vi "Old Helium Fridge Cool-Down - With iTC and Fluke MM.vi"() -> ()   [LabVIEW 2014]
uses:
  <vilib>/Analysis/8numeric.llb/1D Numeric Integration.vi
  <instrlib>/Mercury iXX/Public/Libraries/System/Open/Open System.vi
  <vilib>/express/express shared/transition.llb/Dynamic To Waveform Array.vi
  <vilib>/express/express signal manip/GetorSetDDTAttributes/Set DDT Attributes/SetT0.vi
  <vilib>/express/express shared/transition.llb/Waveform Array To Dynamic.vi
  <vilib>/express/express signal manip/GetorSetDDTAttributes/Set DDT Attributes/Set DDT Properties.xnode
  <vilib>/Analysis/NI_AALPro.lvlib
  <instrlib>/Mercury iXX/Mercury iXX.lvlib
  <instrlib>/Mercury iXX/Public/Libraries/System.lvlib
panel:
  out "Centroid:":dbl
  out "Tri":bool
  out "NMR":bool
  out "NMR":cluster{"Y":dbl[], "Y":dbl[]}[](graph)
  out "AB4.R":dynamicdata(graph)
  out "AB4.T":dynamicdata(graph)
  out "AB3.R":dynamicdata(graph)
  out "AB3.T":dynamicdata(graph)
  out "Fluke Err":bool
  out "Mag. Field (T)":dbl
  in  "Peak Location (MHz)":dbl
  in  "Baseline Subtract":bool
  out "AB2.R":dynamicdata(graph)
  out "AB2.T":dynamicdata(graph)
  out "Peak Location (MHz)":dbl
  in  "Mag. Field (T)":dbl
  out "i":dbl
  in  "VISA resource name":refnum<visa-resource-name>="MERCURYITC"
  in  "Time b/t iTC Resets\n(min)":dbl=45.0
  out "Time Since iTC Reset\n(min)":dbl
  out "iTC Last Reset":timestamp
  out "Reset iTC":bool
  in  "Wing Fit Poly":i32=3 min=0 max=4 step=1
  out "Just Started":bool
  out "Up/Down Ave Y Final":dbl[](array[numeric])
  in  "Use Wing Fit":bool=TRUE
  out "Triangle Wave\nRate (Hz)":dbl
  in  "NMR Temp Points/Measurement":dbl=20.0
  in  "Peak Size":dbl=15.0 min=0.0 max=100.0
  out "Wing Fit":dbl[](array[numeric])
  out "Fit Y":dbl[](array[numeric])
  out "Fit X":dbl[](array[numeric])
  in  "Wing Size (%)":dbl=20.0 min=0.0 max=100.0
  out "Normalized\nAdditive NMR Y":dbl[](array[numeric])
  out "Up/Down Ave Y":dbl[](array[numeric])
  out "Up/Down Ave X":dbl[](array[numeric])
  out "Baseline\nSubtract":bool
  out "Depth/Div Submit":bool
  out "Cent. Frq. Submit":bool
  out "Insta Mod One":dbl[](array[numeric])
  out "Insta Tri":dbl[](array[numeric])
  out "Insta Mod Sweeps":dbl[](array[numeric])
  in  "Triangle Wave Rate\nSubmit":bool
  in  "Session In 3":refnum<visa-resource-name>="HPSIGGEN"
  in  "error in 3":errorcluster {"code" format="%.0x"}
  out "Central Frequency 2":dbl
  out "error out 3":errorcluster {"code" format="%.0x"}
  out "Session Out 3":refnum<visa-resource-name>
  out "Reset Sweep":bool
  out "Add Mod Sweep":dbl[](array[numeric])
  out "Sweep Iter":i32
  out "Array Size":i32
  out "Modulator":dbl[](array[numeric])
  out "Reference Triangle Wave":dbl[](array[numeric])
  out "Input Triangle Wave":dbl[](array[numeric])
  out "Triangle Check":dbl
  out "NMR X Check":dbl[](array[numeric])
  out "NMR":cluster{"Y":dbl[], "Y":dbl[]}[](graph)
  in  "Reset Total\nSweeps":bool
  out "Number of Total\nSweeps Added":i32
  out "Additive NMR Y":dbl[](array[numeric])
  out "Good NMR X":dbl[](array[numeric])
  in  "Record All\nSweep Sets":bool
  out "Flow (SLM)":dbl
  out "NMR":bool
  out "AB   .T":i32
  out "AB":i32
  out "Roots Flow (SLM)":dynamicdata(graph)
  in  "DV4/DV6":bool
  out "Temp":bool
  out "AB5.R":dynamicdata(graph)
  out "CCS.R":dynamicdata(graph)
  out "AB2/3/4.R":dynamicdata(graph)
  out "AB1.R":dynamicdata(graph)
  out "AB5.T":dynamicdata(graph)
  out "CCS.T":dynamicdata(graph)
  out "AB2/3/4.T":dynamicdata(graph)
  out "AB1.T":dynamicdata(graph)
  out "Vapor Pressure\n(mTorr)":dbl
  out "V.P. Voltage\n(V)":dbl
  in  "LN2/LHe":bool=TRUE
  out "V.P. Temp\n(K)":dbl
  out "Vapor Pressure":dynamicdata(graph)
  out "Vapor Pressure\n(mbar)":dbl format="%#_3e"
  out "Vapor Pressure\n(mTorr)":dbl
  in  "Time Between\nTemp Ponts (s)":dbl=5.0
  out "?":dbl
  out "?":dbl
  out "?":dbl
  out "?":dbl
  out "Baseline X":dbl[](array[numeric])
  out "Session Out 2":refnum<visa-resource-name>
  out "error out 2":errorcluster {"code" format="%.0x"}
  out "token":dbl
  in  "error in 2":errorcluster {"code" format="%.0x"}
  in  "Session In 2":refnum<visa-resource-name>="HPSIGGEN"
  in  "Depth/Div Submit":bool
  out "Depth/Div (kHz)":dbl
  in  "Cent. Frq. Submit":bool
  out "Session Out":refnum<visa-resource-name>
  out "error out":errorcluster {"code" format="%.0x"}
  out "Central Frequency":dbl
  in  "error in":errorcluster {"code" format="%.0x"}
  in  "Session In":refnum<visa-resource-name>="HPSIGGEN"
  out "Cent. Freq. (MHz)":dbl
  out "Temp":bool
  out "Temperature Strip Chart":dynamicdata(graph)
  out "Q Meter Temp":dynamicdata(graph)
  out "Zeroed Array":dbl[](array[numeric])
  in  "Submit":bool
  out "Is Flashing":bool
  in  "Error Beat":bool
  in  "Clear":bool
  in  "Comment":string
  out "Heartbeat":bool
  out "Most Recent Error":string
  out "Baseline Subtracted Integral vs. Time":dbl(graph)
  out "Time of Last Baseline":string
  out "Baseline Y":dbl[](array[numeric])
  in  "Get Baseline":bool
  out "Recording":bool
  out "Time of Last Recording":string
  in  "Record Next \nSweep Set":bool
  in  "Depth/Div\n(MHz)":dbl=0.5
  in  "Central Freq. \n(MHz)":dbl=12.996
  in  "Triangle Wave\nRate (Hz)":dbl=15.862
  out "Time Elapsed \nDuring Sweeps (s)":dbl
  out "Lab Time":string
  out "Most Recent Error (NMR)":string
  out "Last Sweep Start Time":string
  out "Most Recent Error (Temp)":string
  out "Last Measurement Taken":string
  out "VI Start Time":string
  out "Temp":bool
  out "NMR":bool
  in  "stop":bool
  out "Input Triangle Wave":dynamicdata(graph)
  out "Modulator":dynamicdata(graph)
  in  "# of Sweeps":i32=1
  out "Resistance Strip Chart":dynamicdata(graph)
  in  "Heartbeat":bool
  in  "Temp Strip Chart":bool
  out "Errors":bool
  in  "Silence Flashing":bool
  in  "Ignore \nErrors":bool
  out "NMR":cluster{"Y":dbl[], "Y":dbl[]}[](graph)
  in  "AB2/3/4 Switch":T1(radio)=enum."Radio Selection 3"
  # "Initialization and Logic Controls -- DO NOT TOUCH!!"
  # "Signal Generator Logic -- DO NOT TOUCH!!"
  # "To Clean and Get Rid Of"
  # "Baseline = 3000 Sweeps"
  # "TE > 2000 Sweeps"
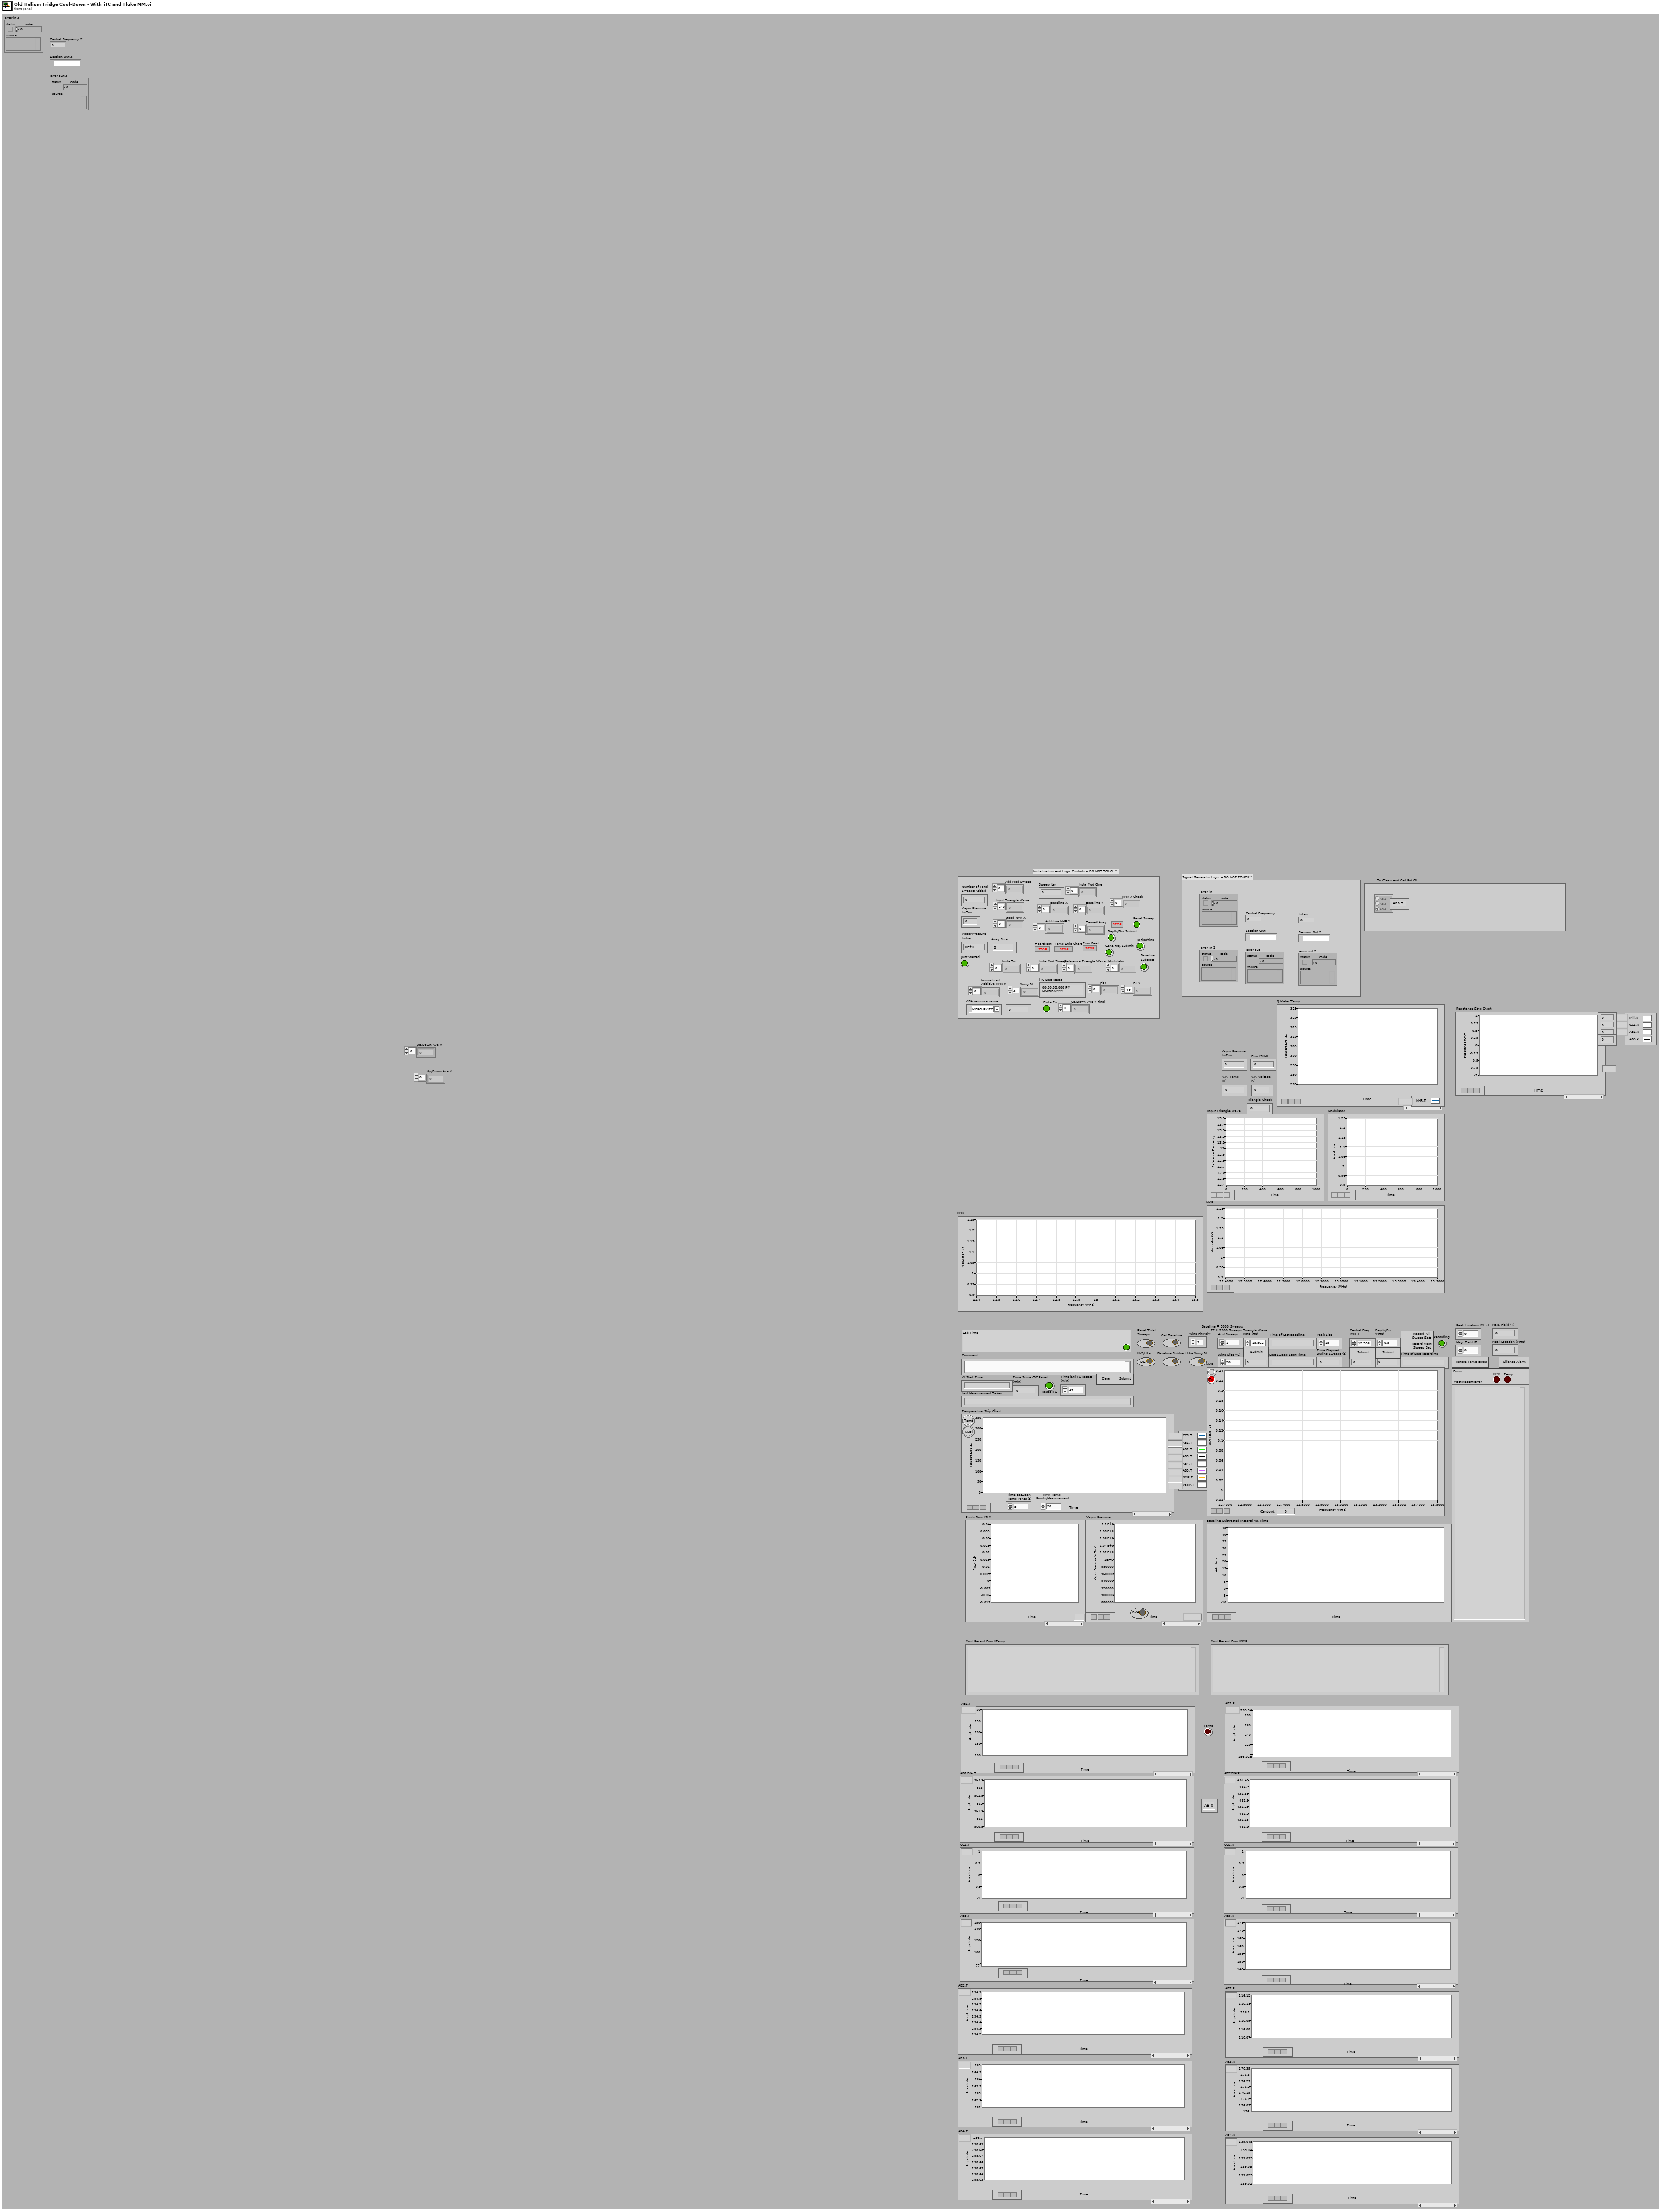
[diagram p1: front panel]
types:
  T1 = enum32{"Radio Selection 1", "Radio Selection 2", "Radio Selection 3"}
  T2 = typedef "Mercury iXX.lvlib/Mercury Reference.ctl" = cluster{"Comms":refnum<visa-resource-name>, "Device ID":string[], "Comms Layer":T3, "Command":string, "Query reference":T4}
  T3 = typedef "Mercury iXX.lvlib/Comms Transport Layer.ctl" = enum16{"Ethernet TCP/IP", "USB", "ISOBus - RS-232", "GPIB"}
  T4 = typedef "Mercury iXX.lvlib/Query Dynamic Reference.ctl" = refnum<vi>
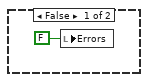
[diagram p2: hidden frame]
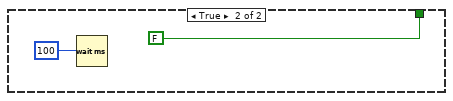
[diagram p4: hidden frame]
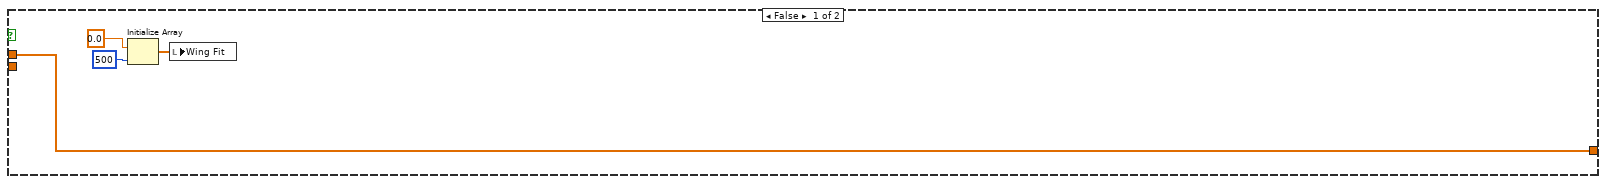
[diagram p6: hidden frame]
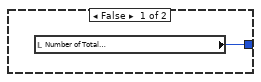
[diagram p8: hidden frame]
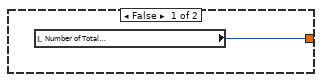
[diagram p10: hidden frame]
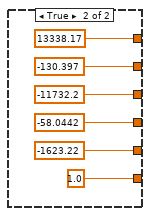
[diagram p11: hidden frame]
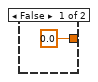
[diagram p12: hidden frame]
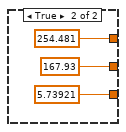
[diagram p13: hidden frame]
diagram:
  # "Initialize Baseline to All Zeros"
  n1 = while "NMR System" {
    stop <- "stop" stop-if-true
    w78 = 490
    w86 = 0
    w74 = 2.0
    w77 = 500
    n2 = local read "Just Started"() -> (w33:bool)
    n3 = local read "Just Started"() -> (w36:bool)
    n4 = local read "Just Started"() -> (w28:bool)
    n5 = local read "Central Frequency"() -> (w155:dbl)
    n6 = Get Date/Time In Seconds() -> (seconds since 1Jan1904=w171:timestamp)
    n7 = Or(x="Cent. Frq. Submit", y=w36) -> (x .or. y?=w34:bool)
    "Cent. Frq. Submit" <- w34
    n8 = Or(x="Triangle Wave Rate\nSubmit", y=w33) -> (x .or. y?=w31:bool)
    n9 = Or(x="Depth/Div Submit", y=w28) -> (x .or. y?=w29:bool)
    "Depth/Div Submit" <- w29
    n10 = Get Date/Time String(seconds (now)=w171, want seconds? (F)=TRUE) -> (date string=w174:string, time string=w176:string)  [unwired: 1 in]
    n11 = case "Set Central Frequency" shown="True" w34 {
      tunnel: "Central Freq. \n(MHz)" -> [_ w353]
      frame False {
      }
      frame True {
        w351 = " MHz; FREQuency:CW?"  # Command
        w354 = "FREQuency "  # Command
        w372 = "[,;\r\n\t]+"  # Delimiters
        w369 = "%.;%f"  # Format String
        (unwired) "FREQuency 12.996 MHz; FREQuency:CW?"  # Command
        w360 = u8 0  # Termination Char
        w355 = u32 3000  # Timeout
        # "Parse the output text based on the Format String"
        # "Perform a VISA Write and Read (Query)"
        # "Keep reading 4096 bytes while the error returned from the\nVISA read 0x3FFF0006 (there's more data in the buffer to read)."
        # "Set the termination character"
        n12 = property class="Instr"(reference="Session In", error in="error in", "General Settings:Timeout Value"=w355) -> (reference out=w361:refnum<visa-resource-name>, error out=w358:errorcluster)
        n13 = property class="Instr"(reference=w361, error in=w358, "Message Based Settings:Termination Character"=w360, "Message Based Settings:Termination Character Enable"=FALSE ("enable")) -> (reference out=w373:refnum<visa-resource-name>, error out=w359:errorcluster)
        "Session Out" <- w373
        n14 = Number To Fractional String(number=w353) -> (F-format string=w352:string)  [unwired: 3 in]
        n15 = Concatenate Strings(w354, w352, w351) -> (w350:string)
        n16 = VISA Write(VISA resource name=w373, write buffer=w350, error in (no error)=w359) -> (VISA resource name out=w363:refnum<visa-resource-name>, error out=w364:errorcluster)  [unwired: 1 out]
        n17 = while {
          tunnel: w363 -> [w380]
          shift-right: [w374] -> w367
          shift-left: "" -> [w379]
          tunnel: w364 -> [w377]
          tunnel: [w376] -> w365
          stop <- w375 continue-if-true
          n18 = VISA Read(VISA resource name=w380, byte count=u32 4096 ("byte count (0)"), error in (no error)=w377) -> (read buffer=w378:string, error out=w376:errorcluster)  [unwired: 2 out]
          n19 = Unbundle By Name(w376) -> ("code"=w382:i32)
          n20 = Concatenate Strings(w379, w378) -> (w374:string)
          n21 = Equal?(x=1073676294, y=w382) -> (x = y?=w375:bool)
        }
        n22 = Match Pattern(string=w367, regular expression=w372) -> (before substring=w368:string)  [unwired: 1 in, 3 out]
        n23 = Scan From String(format string=w369, input string=w368, error in=w365) -> (error out=→"error out":errorcluster, output 1=→"Central Frequency":dbl)  [unwired: 2 in, 2 out]
      }
    }
    n24 = case "Set Triangle Wave Frequency" shown="True" w31 {
      tunnel: "Triangle Wave\nRate (Hz)" -> [_ w235]
      frame False {
      }
      frame True {
        w237 = " Hz; FM1:INTernal:FREQuency?"  # Command
        w239 = "FM1:INTernal1:FREQuency "  # Command
        w256 = "[,;\r\n\t]+"  # Delimiters
        w254 = "%.;%f"  # Format String
        (unwired) "FM1:INTernal1:FREQuency 15 Hz; FM1:INTernal:FREQuency?"  # Command
        w245 = u8 0  # Termination Char
        w240 = u32 3000  # Timeout
        # "Parse the output text based on the Format String"
        # "Perform a VISA Write and Read (Query)"
        # "Keep reading 4096 bytes while the error returned from the\nVISA read 0x3FFF0006 (there's more data in the buffer to read)."
        # "Set the termination character"
        n25 = property class="Instr"(reference="Session In 3", error in="error in 3", "General Settings:Timeout Value"=w240) -> (reference out=w246:refnum<visa-resource-name>, error out=w243:errorcluster)
        n26 = property class="Instr"(reference=w246, error in=w243, "Message Based Settings:Termination Character"=w245, "Message Based Settings:Termination Character Enable"=FALSE ("enable")) -> (reference out=w257:refnum<visa-resource-name>, error out=w244:errorcluster)
        "Session Out 3" <- w257
        n27 = Number To Fractional String(number=w235) -> (F-format string=w238:string)  [unwired: 3 in]
        n28 = Concatenate Strings(w239, w238, w237) -> (w236:string)
        n29 = VISA Write(VISA resource name=w257, write buffer=w236, error in (no error)=w244) -> (VISA resource name out=w248:refnum<visa-resource-name>, error out=w249:errorcluster)  [unwired: 1 out]
        n30 = while {
          tunnel: w248 -> [w264]
          shift-right: [w258] -> w252
          shift-left: "" -> [w263]
          tunnel: w249 -> [w261]
          tunnel: [w260] -> w250
          stop <- w259 continue-if-true
          n31 = VISA Read(VISA resource name=w264, byte count=u32 4096 ("byte count (0)"), error in (no error)=w261) -> (read buffer=w262:string, error out=w260:errorcluster)  [unwired: 2 out]
          n32 = Unbundle By Name(w260) -> ("code"=w266:i32)
          n33 = Concatenate Strings(w263, w262) -> (w258:string)
          n34 = Equal?(x=1073676294, y=w266) -> (x = y?=w259:bool)
        }
        n35 = Match Pattern(string=w252, regular expression=w256) -> (before substring=w253:string)  [unwired: 1 in, 3 out]
        n36 = Scan From String(format string=w254, input string=w253, error in=w250) -> (error out=→"error out 3":errorcluster, output 1=→"Central Frequency 2":dbl)  [unwired: 2 in, 2 out]
        "Triangle Wave\nRate (Hz)" <- w235
      }
    }
    n37 = local read "token"() -> (w152:dbl)
    n38 = case "Set Depth/Div" shown="True" w29 {
      tunnel: "Depth/Div\n(MHz)" -> [_ w315]
      frame False {
      }
      frame True {
        w317 = " Hz; :FM1:DEViation?"  # Command
        w322 = "[,;\r\n\t]+"  # Delimiters
        w325 = "%.;%f"  # Format String
        w319 = ":FM1:DEViation "  # Command
        w334 = u8 0  # Termination Char
        w339 = u32 3000  # Timeout
        # "Parse the output text based on the Format String"
        # "Perform a VISA Write and Read (Query)"
        # "Keep reading 4096 bytes while the error returned from the\nVISA read 0x3FFF0006 (there's more data in the buffer to read)."
        # "Set the termination character"
        n39 = property class="Instr"(reference="Session In 2", error in="error in 2", "General Settings:Timeout Value"=w339) -> (reference out=w333:refnum<visa-resource-name>, error out=w336:errorcluster)
        n40 = Multiply(x=w315, y=1000000.0) -> (x*y=w314:dbl)
        n41 = property class="Instr"(reference=w333, error in=w336, "Message Based Settings:Termination Character"=w334, "Message Based Settings:Termination Character Enable"=FALSE ("enable")) -> (reference out=w321:refnum<visa-resource-name>, error out=w335:errorcluster)
        "Session Out 2" <- w321
        n42 = Number To Fractional String(number=w314) -> (F-format string=w318:string)  [unwired: 3 in]
        n43 = Concatenate Strings(w319, w318, w317) -> (w320:string)
        n44 = VISA Write(VISA resource name=w321, write buffer=w320, error in (no error)=w335) -> (VISA resource name out=w331:refnum<visa-resource-name>, error out=w330:errorcluster)  [unwired: 1 out]
        n45 = while {
          tunnel: w331 -> [w346]
          shift-right: [w340] -> w327
          shift-left: "" -> [w345]
          tunnel: w330 -> [w343]
          tunnel: [w342] -> w329
          stop <- w341 continue-if-true
          n46 = VISA Read(VISA resource name=w346, byte count=u32 4096 ("byte count (0)"), error in (no error)=w343) -> (read buffer=w344:string, error out=w342:errorcluster)  [unwired: 2 out]
          n47 = Unbundle By Name(w342) -> ("code"=w348:i32)
          n48 = Concatenate Strings(w345, w344) -> (w340:string)
          n49 = Equal?(x=1073676294, y=w348) -> (x = y?=w341:bool)
        }
        n50 = Match Pattern(string=w327, regular expression=w322) -> (before substring=w326:string)  [unwired: 1 in, 3 out]
        n51 = Scan From String(format string=w325, input string=w326, error in=w329) -> (error out=→"error out 2":errorcluster, output 1=→"token":dbl)  [unwired: 2 in, 2 out]
      }
    }
    n52 = Concatenate Strings(w174, " ", w176) -> (w166:string)
    n53 = Divide(x=w155, y=1000000.0) -> (x/y=w154:dbl)
    "Cent. Freq. (MHz)" <- w154
    n54 = Divide(x=w152, y=1000000.0) -> (x/y=w151:dbl)
    "Depth/Div (kHz)" <- w151
    n55 = while "Sweep-Averaged Modulator and Triangle Input" {
      tunnel: "# of Sweeps" -> [w585]
      tunnel: 1000 -> [w555]
      tunnel: [w568] -> w93
      tunnel: w166 -> [w595]
      tunnel: [w594] -> w172
      tunnel: [w593] -> w169
      tunnel: w151 -> [w589]
      tunnel: w154 -> [w587]
      tunnel: [w586] -> w94
      tunnel: [w580] -> w158
      tunnel: [w575] -> w140
      tunnel: [w569] -> w103
      i -> [w570]
      stop <- w556 stop-if-true
      w550 = 42.57
      w583 = 0.0
      n56 = local read "Reset Sweep"() -> (w557:bool)
      n57 = local read "Sweep Iter"() -> (w560:i32)
      n58 = Greater Or Equal?(x=w570, y=w585) -> (x >= y?=w558:bool)
      n59 = Equal To 0?(x=w570) -> (x = 0?=w564:bool)
      n60 = local read "Triangle Wave\nRate (Hz)"() -> (w554:dbl)
      n61 = Multiply(x="Mag. Field (T)", y=w550) -> (x*y=→"Peak Location (MHz)":dbl)
      n62 = Not Equal To 0?(x=w560) -> (x != 0?=w561:bool)
      n63 = case shown="True" w564 {
        frame False {
        }
        frame True {
          "Sweep Iter" <- 0
        }
      }
      n64 = Compound Arithmetic op=OR(w558, w557) -> (w556:bool)
      n65 = Divide(x="Peak Location (MHz)", y=w550) -> (x/y=→"Mag. Field (T)":dbl)
      n66 = case shown="True" w561 {
        frame False {
        }
        frame True {
          n67 = control-ref of="Reference Triangle Wave"() -> (w613:refnum<vi>)
          n68 = local read "Baseline\nSubtract"() -> (w608:bool)
          n69 = control-ref of="Insta Mod Sweeps"() -> (w615:refnum<vi>)
          n70 = control-ref of="Number of Total\nSweeps Added"() -> (w606:refnum<vi>)
          n71 = control-ref of="Up/Down Ave X"() -> (w602:refnum<vi>)
          n72 = control-ref of="Normalized\nAdditive NMR Y"() -> (w607:refnum<vi>)
          n73 = control-ref of="Insta Mod One"() -> (w609:refnum<vi>)
          n74 = control-ref of="Baseline X"() -> (w610:refnum<vi>)
          n75 = control-ref of="Baseline Y"() -> (w611:refnum<vi>)
          n76 = control-ref of="Sweep Iter"() -> (w612:refnum<vi>)
          n77 = control-ref of="Insta Tri"() -> (w614:refnum<vi>)
          n78 = control-ref of="Fit X"() -> (w605:refnum<vi>)
          n79 = control-ref of="Fit Y"() -> (w604:refnum<vi>)
          n80 = control-ref of="Wing Fit"() -> (w603:refnum<vi>)
          n81 = control-ref of="Up/Down Ave Y"() -> (w601:refnum<vi>)
          n82 = call "Baseline Monitor.vi"("Baseline X"=w610, "Baseline Y"=w611, "Sweep Iter"=w612, "Reference Triangle Wave"=w613, "Input Triangle Wave"=w614, "Modulator"=w615, "Insta Mod"=w609, "Normalized\nAdditive NMR\nY"=w607, "Baseline\nSubtract"=w608, "Wings X"=w605, "# of Sweeps"=w606, "Wings Y"=w604, "Wing Fit"=w603, "Up/Down Ave X"=w602, "Up/Down Ave Y"=w601) -> ()  [unwired: 5 in]
        }
      }
      n83 = To Double Precision Float(number=w555) -> (double precision float=w592:dbl)
      n84 = Multiply(x=w554, y=w592) -> (x*y=w553:dbl)
      n85 = call "Get NMR Data"("rate"=w553, "number of samples"=w555) -> ("data"=w600:dynamicdata, "error out"=w575:errorcluster)  [unwired: 15 in, 1 out]
      n86 = while {
        tunnel: ["NMR Temp Points/Measurement"] -> w578
        tunnel: [w646] -> w577
        tunnel: w575 -> [w642]
        i -> [w645]
        stop <- w644 stop-if-true
        n87 = call "Get NMR Temp"("error in"=w642) -> ("data"=w648:dynamicdata)  [unwired: 16 in, 2 out]
        n88 = Add(x=w648, y=273.15) -> (x+y=w647:dynamicdata)
        n89 = call "Convert from Dynamic Data7"("Dynamic Data Type"=w647) -> ("Scalar"=w650:dbl)  [unwired: 3 in]
        n90 = Equal To 0?(x=w645) -> (x = 0?=w651:bool)
        n91 = Greater Or Equal?(x=w645, y="NMR Temp Points/Measurement") -> (x >= y?=w644:bool)
        n92 = feedback #1() -> (w653:dbl)  [unwired: 1 in]
        n93 = Add(x=w650, y=w653) -> (x+y=w646:dbl)
        n94 = Select(t=0.0, s=w651, f=w646) -> (s? t:f=w652:dbl)
        n95 = feedback-in #1(w652) -> ()
      }
      n96 = Split Signals(w600) -> (w591:dynamicdata, w599:dynamicdata)  [unwired: 2 in]
      n97 = call <vilib>:"General Error Handler.vi"("type of dialog (OK msg:1)"=0, "error in (no error)"=w575) -> ("error?"=w579:bool, "message"=w597:string, "error out"=w593:errorcluster)  [unwired: 9 in, 2 out]
      "NMR" <- w579
      "NMR" <- w579
      n98 = call "Convert from Dynamic Data2"("Dynamic Data Type"=w591) -> ("Array"=w590:dbl[])  [unwired: 3 in]
      n99 = call "Convert from Dynamic Data"("Dynamic Data Type"=w599) -> ("Array"=w559:dbl[])  [unwired: 3 in]
      "Insta Mod One" <- w559
      n100 = case shown="False" w579 {
        tunnel: w597 -> [_ w657]
        tunnel: w595 -> [w655 _]
        frame False {
          "Last Sweep Start Time" <- w655
        }
        frame True {
          n101 = local read "Lab Time"() -> (w659:string)
          n102 = Concatenate Strings(w659, "; ", w657) -> (→"Most Recent Error (NMR)":string)
        }
      }
      n103 = Multiply(x=w590, y=w589) -> (x*y=w588:dbl[])
      n104 = Add(x=w588, y=w587) -> (x+y=w562:dbl[])
      "Insta Tri" <- w562
      n105 = local read "Good NMR X"() -> (w574:dbl[])
      n106 = while {
        tunnel: w562 -> [w627]
        tunnel: w574 -> [w626]
        tunnel: [w624] -> w572
        i -> [w623]
        stop <- w637 stop-if-true
        n107 = Array Size(array=w627) -> (size(s)=w624:i32)
        n108 = Greater Or Equal?(x=w623, y=w624) -> (x >= y?=w637:bool)
        n109 = Equal To 0?(x=w623) -> (x = 0?=w630:bool)
        n110 = Index Array(array=w626, index=w623) -> (element=w625:dbl)
        n111 = case shown="True" w630 {
          frame False {
          }
          frame True {
            "Triangle Check" <- 0.0
          }
        }
        n112 = Multiply(x=0.01, y=w625) -> (x*y=w634:dbl)
        n113 = Add(x=w634, y=w625) -> (x+y=w635:dbl)
        n114 = Subtract(x=w625, y=w634) -> (x-y=w633:dbl)
        n115 = Index Array(array=w627, index=w623) -> (element=w628:dbl)
        n116 = Less?(x=w628, y=w635) -> (x < y?=w632:bool)
        n117 = Greater?(x=w628, y=w633) -> (0:w631:bool)
        n118 = And(x=w632, y=w631) -> (x .and. y?=w629:bool)
        n119 = case shown="True" w629 {
          frame False {
          }
          frame True {
            n120 = local read "Triangle Check"() -> (w639:dbl)
            n121 = Add(x=1.0, y=w639) -> (x+y=w640:dbl)
            n122 = local write "Triangle Check"(w640) -> ()
          }
        }
      }
      "Array Size" <- w572
      n123 = call "Convert to Dynamic Data10"("Array"=w562) -> ("Dynamic Data Type"=w586:dynamicdata)  [unwired: 3 in]
      n124 = local read "Sweep Iter"() -> (w569:i32)
      n125 = Divide(x=w577, y=w578) -> (x/y=w576:dbl)
      n126 = local read "Add Mod Sweep"() -> (w565:dbl[])
      n127 = Initialize Array(w583, w555) -> (w598:dbl[])
      n128 = Equal To 0?(x=w569) -> (x = 0?=w584:bool)
      n129 = local read "Sweep Iter"() -> (w566:i32)
      n130 = Select(t=w598, s=w584, f=w565) -> (s? t:f=w567:dbl[])
      "Add Mod Sweep" <- w567
      n131 = feedback #2() -> (w581:dbl)  [unwired: 1 in]
      n132 = Add(x=w576, y=w581) -> (x+y=w580:dbl)
      n133 = Select(t=w583, s=w584, f=w580) -> (s? t:f=w582:dbl)
      n134 = feedback-in #2(w582) -> ()
      n135 = Divide(x=w567, y=w566) -> (x/y=→"Insta Mod Sweeps":dbl[])
      n136 = local read "Triangle Check"() -> (w573:dbl)
      n137 = Equal?(x=w573, y=w572) -> (x = y?=w571:bool)
      "Tri" <- w571
      n138 = case shown="True" w571 {
        tunnel: w559 -> [_ w620]
        frame False {
        }
        frame True {
          n139 = local read "Sweep Iter"() -> (w618:i32)
          n140 = local read "Add Mod Sweep"() -> (w621:dbl[])
          n141 = Add(x=w618, y=1) -> (x+y=w616:i32)
          n142 = Add(x=w621, y=w620) -> (x+y=w619:dbl[])
          n143 = local write "Sweep Iter"(w616) -> ()
          n144 = local write "Add Mod Sweep"(w619) -> ()
        }
      }
      n145 = local read "Add Mod Sweep"() -> (w568:dbl[])
      n146 = Get Date/Time In Seconds() -> (seconds since 1Jan1904=w594:timestamp)
    }
    n147 = local read "Good NMR X"() -> (w110:dbl[])
    n148 = local read "Depth/Div Submit"() -> (w98:bool)
    n149 = local read "Cent. Frq. Submit"() -> (w99:bool)
    n150 = local read "Just Started"() -> (w37:bool)
    n151 = call "Convert to Dynamic Data33"("Array"=w110) -> ("Dynamic Data Type"=w105:dynamicdata)  [unwired: 3 in]
    n152 = call "DAQ Assistant"("error in"=w140) -> ("data"=w146:dynamicdata, "error out"=w130:errorcluster)  [unwired: 16 in, 1 out]
    n153 = case shown="False" "DV4/DV6" {
      tunnel: [9.563177 13338.17] -> w139
      tunnel: [-6.30995 -130.397] -> w138
      tunnel: [-4.4943 -11732.2] -> w137
      tunnel: [-6.91233 -58.0442] -> w136
      tunnel: [-5.10184 -1623.22] -> w135
      tunnel: [1000.0 1.0] -> w133
      frame False {
      }
      frame True {
      }
    }
    n154 = case shown="False" w37 {
      selector: w37 -> [w179 _]
      tunnel: [w179 FALSE] -> w27
      frame False {
      }
      frame True {
        n155 = Wait (ms)(milliseconds to wait=100) -> ()  [unwired: 1 out]
      }
    }
    n156 = Subtract(x=w172, y=w171) -> (x-y=→"Time Elapsed \nDuring Sweeps (s)":dbl)
    n157 = Merge Signals(w94, w105) -> (→"Input Triangle Wave":dynamicdata)
    n158 = call "Convert from Dynamic Data9"("Dynamic Data Type"=w105) -> ("Array"=→"Reference Triangle Wave":dbl[])  [unwired: 3 in]
    n159 = Compound Arithmetic op=OR(w37, "Reset Total\nSweeps", w99, w98) -> (w100:bool)
    "Reset Sweep" <- w100
    n160 = call "Convert from Dynamic Data8"("Dynamic Data Type"=w94) -> ("Array"=w107:dbl[])  [unwired: 3 in]
    "Input Triangle Wave" <- w107
    n161 = Divide(x=w93, y=w103) -> (x/y=w68:dbl[])
    "Modulator" <- w68
    n162 = Divide(x=w158, y=w103) -> (x/y=w159:dbl)
    n163 = local read "Tri"() -> (w104:bool)
    n164 = case shown="True" w104 {
      tunnel: w93 -> [_ w272]
      tunnel: [w268 w270] -> w109
      tunnel: w103 -> [_ w269]
      frame False {
        n165 = local read "Number of Total\nSweeps Added"() -> (w268:i32)
      }
      frame True {
        n166 = local read "Additive NMR Y"() -> (w274:dbl[])
        n167 = local read "Number of Total\nSweeps Added"() -> (w271:i32)
        n168 = Add(x=w272, y=w274) -> (x+y=w273:dbl[])
        n169 = local write "Additive NMR Y"(w273) -> ()
        n170 = Add(x=w271, y=w269) -> (x+y=w270:i32)
      }
    }
    "Number of Total\nSweeps Added" <- w109
    n171 = case shown="True" w100 {
      tunnel: w107 -> [_ w275]
      frame False {
      }
      frame True {
        n172 = local write "Good NMR X"(w275) -> ()
      }
    }
    n173 = case shown="True" w100 {
      tunnel: [w276 0.0] -> w64
      frame False {
        n174 = local read "Number of Total\nSweeps Added"() -> (w276:i32)
      }
      frame True {
        n175 = Initialize Array(0.0, 1000) -> (w277:dbl[])
        n176 = local write "Good NMR X"(w277) -> ()
        n177 = local write "Additive NMR Y"(w277) -> ()
      }
    }
    n178 = call "DAQ Assistant2"("error in"=w130) -> ("data"=w129:dynamicdata)  [unwired: 16 in, 2 out]
    n179 = local read "Baseline Y"() -> (w79:dbl[])
    n180 = Add(x=w78, y=w77) -> (x+y=w85:i32)
    n181 = Greater Than 0?(x=w159) -> (x > 0?=w165:bool)
    n182 = To Double Precision Float(number=w146) -> (double precision float=w141:dbl)
    "V.P. Voltage\n(V)" <- w141
    n183 = Less?(x=w159, y=500.0) -> (x < y?=w162:bool)
    n184 = To Double Precision Float(number=w129) -> (double precision float=w128:dbl)
    n185 = Array Subset(array=w68, index=w78, length=w77) -> (w97:dbl[])
    n186 = Array Subset(array=w68, index=w85, length=w77) -> (w90:dbl[])
    n187 = call "Convert to Dynamic Data9"("Array"=w68) -> ("Dynamic Data Type"=w112:dynamicdata)  [unwired: 3 in]
    n188 = Array Subset(array=w79, index=w85, length=w77) -> (w84:dbl[])
    n189 = And(x=w162, y=w165) -> (x .and. y?=w164:bool)
    n190 = call "Convert to Dynamic Data15"("Double"=w159) -> ("Dynamic Data Type"=w160:dynamicdata)  [unwired: 3 in]
    n191 = Greater?(x=w141, y=0.049) -> (0:w145:bool)
    n192 = case "Take Baseline Structure" shown="True" "Get Baseline" {
      tunnel: w112 -> [_ w393]
      tunnel: w166 -> [_ w394]
      tunnel: w94 -> [_ w391]
      frame False {
      }
      frame True {
        n193 = call "Convert from Dynamic Data4"("Dynamic Data Type"=w393) -> ("Array"=w395:dbl[])  [unwired: 3 in]
        n194 = call "Convert from Dynamic Data6"("Dynamic Data Type"=w391) -> ("Array"=w392:dbl[])  [unwired: 3 in]
        n195 = local write "Baseline Y"(w395) -> ()
        n196 = local write "Baseline X"(w392) -> ()
        "Time of Last Baseline" <- w394
      }
    }
    n197 = case shown="True" w164 {
      tunnel: w160 -> [_ w384]
      frame False {
      }
      frame True {
        "Q Meter Temp" <- w384
      }
    }
    n198 = formula code="P=(a+c*V+e*V*V)/(1+b*V+d*V*V);"("V"=w141, "a"=w135, "b"=w136, "c"=w137, "d"=w138, "e"=w139) -> ("P"=w143:dbl)
    n199 = local write "Just Started"(w27) -> ()
    n200 = Array Size(array=w90) -> (size(s)=w89:i32)
    n201 = Array Subset(array=w68, index=w86, length=w78) -> (w92:dbl[])
    n202 = Array Size(array=w84) -> (size(s)=w83:i32)
    n203 = Array Subset(array=w79, index=w86, length=w78) -> (w82:dbl[])
    n204 = Not(x=w164) -> (.not. x?=→"NMR":bool)
    n205 = Multiply(x=w128, y=10.0) -> (x*y=w126:dbl)
    "Flow (SLM)" <- w126
    n206 = Insert Into Array(array=w90, index=w89, new element=w92) -> (w91:dbl[])
    n207 = Insert Into Array(array=w84, index=w83, new element=w82) -> (w81:dbl[])
    n208 = call "Convert to Dynamic Data20"("Double"=w126) -> ("Dynamic Data Type"=→"Roots Flow (SLM)":dynamicdata)  [unwired: 3 in]
    n209 = Select(t=w143, s=w145, f=999.999) -> (s? t:f=w132:dbl)
    n210 = Array Subset(array=w79, index=w78, length=w77) -> (w76:dbl[])
    n211 = Reverse 1D Array(array=w91) -> (reversed array=w96:dbl[])
    n212 = Reverse 1D Array(array=w81) -> (reversed array=w80:dbl[])
    n213 = Add(x=w97, y=w96) -> (x+y=w95:dbl[])
    n214 = Add(x=w76, y=w80) -> (x+y=w75:dbl[])
    n215 = Multiply(x=w132, y=w133) -> (x*y=w131:dbl)
    "Vapor Pressure\n(mTorr)" <- w131
    "Vapor Pressure\n(mTorr)" <- w131
    n216 = local read "Baseline Subtract"() -> (w71:bool)
    n217 = Multiply(x=w131, y=0.0013332237) -> (x*y=→"Vapor Pressure\n(mbar)":dbl)
    n218 = Divide(x=w75, y=w74) -> (x/y=w73:dbl[])
    n219 = Divide(x=w95, y=w74) -> (x/y=w69:dbl[])
    n220 = local read "Additive NMR Y"() -> (w117:dbl[])
    n221 = case shown="True" "LN2/LHe" {
      tunnel: [0.0 w295] -> w149
      tunnel: w131 -> [_ w294]
      frame False {
      }
      frame True {
        n222 = Multiply(x=0.001, y=w294) -> (x*y=w296:dbl)
        n223 = Greater?(x=w296, y=-218.0) -> (0:w305:bool)
        n224 = Less?(x=w296, y=-195.0) -> (x < y?=w304:bool)
        n225 = And(x=w305, y=w304) -> (x .and. y?=w302:bool)
        n226 = case shown="False" w302 {
          tunnel: [6.93878 5.73921] -> w299
          tunnel: [330.16 167.93] -> w298
          tunnel: [277.196 254.481] -> w297
          frame False {
          }
          frame True {
          }
        }
        n227 = formula code="T=(B/(A-log(P)))-C;"("A"=w299, "B"=w298, "C"=w297, "P"=w296) -> ("T"=w301:dbl)
        n228 = Add(x=w301, y=273.15) -> (x+y=w295:dbl)
      }
    }
    "V.P. Temp\n(K)" <- w149
    n229 = Subtract(x=w69, y=w73) -> (x-y=w70:dbl[])
    n230 = case shown="True" w71 {
      tunnel: w70 -> [_ w191]
      tunnel: w69 -> [w189 _]
      tunnel: [w189 w191] -> w39
      frame False {
        n231 = Initialize Array(0.0, 500) -> (w186:dbl[])
        n232 = local write "Wing Fit"(w186) -> ()
      }
      frame True {
        (unwired) 3
        w194 = 500
        n233 = Divide(x="Wing Size (%)", y=200.0) -> (x/y=w212:dbl)
        n234 = local read "Up/Down Ave X"() -> (w192:dbl[])
        n235 = Multiply(x=500.0, y=w212) -> (x*y=w199:dbl)
        n236 = To Long Integer(number=w199) -> (32bit integer=w201:i32)
        n237 = To Long Integer(number=w199) -> (32bit integer=w206:i32)
        n238 = Subtract(x=w194, y=w201) -> (x-y=w203:i32)
        n239 = Initialize Array(0.0, w194) -> (→"Wing Fit":dbl[])
        n240 = Subtract(x=500, y=w206) -> (x-y=w208:i32)
        n241 = Array Subset(array=w191, index=0, length=w201) -> (w202:dbl[])
        n242 = Array Subset(array=w191, index=w203, length=w201) -> (w200:dbl[])
        n243 = Array Subset(array=w192, index=0, length=w206) -> (w207:dbl[])
        n244 = Array Subset(array=w192, index=w208, length=w206) -> (w205:dbl[])
        n245 = Insert Into Array(array=w202, index=w201, new element=w200) -> (w197:dbl[])
        "Fit Y" <- w197
        n246 = Insert Into Array(array=w207, index=w206, new element=w205) -> (w198:dbl[])
        "Fit X" <- w198
        n247 = call "Convert to Dynamic Data37"("Array"=w198) -> ()  [unwired: 3 in, 1 out]
        n248 = call <vilib>:"General Polynomial Fit.vi"("Y"=w197, "polynomial order"="Wing Fit Poly", "X"=w198) -> ("Polynomial Coefficients"=w195:dbl[])  [unwired: 9 in, 3 out]
        n249 = while {
          tunnel: w195 -> [w215]
          tunnel: w194 -> [w226]
          tunnel: w192 -> [w221]
          i -> [w224]
          stop <- w225 stop-if-true
          n250 = Index Array(array=w221, index=w224) -> (element=w220:dbl)
          n251 = Greater Or Equal?(x=w224, y=w226) -> (x >= y?=w225:bool)
          n252 = Index Array(array=w215, index=4) -> (element=w216:dbl)
          n253 = Index Array(array=w215, index=3) -> (element=w218:dbl)
          n254 = Index Array(array=w215, index=2) -> (element=w228:dbl)
          n255 = Index Array(array=w215, index=1) -> (element=w229:dbl)
          n256 = Index Array(array=w215, index=0) -> (element=w230:dbl)
          n257 = formula code="y=c0+c1*x+c2*x*x+c3*x*x*x+c4*x*x*x*x;"("x"=w220, "c0"=w230, "c1"=w229, "c2"=w228, "c3"=w218, "c4"=w216) -> ("y"=w233:dbl)
          n258 = local read "Wing Fit"() -> (w223:dbl[])
          n259 = Insert Into Array(array=w223, index=w224, new element=w233) -> (w222:dbl[])
          n260 = local write "Wing Fit"(w222) -> ()
        }
      }
    }
    "Up/Down Ave Y" <- w39
    n261 = To Long Integer(number=w64) -> (32bit integer=w63:i32)
    n262 = local write "Number of Total\nSweeps Added"(w63) -> ()
    n263 = Divide(x=w117, y=w109) -> (x/y=w66:dbl[])
    "Normalized\nAdditive NMR Y" <- w66
    n264 = case "Subtract Baseline" shown="True" "Baseline Subtract" {
      tunnel: w66 -> [w385 w390]
      tunnel: [w385 w387] -> w113
      tunnel: [w385 w387] -> w67
      frame False {
      }
      frame True {
        n265 = local read "Up/Down Ave Y Final"() -> (w386:dbl[])
        n266 = call-poly <vilib>:"Numeric Integration.vi"("Input Array"=w386) -> ("result"=→"Baseline Subtracted Integral vs. Time":dbl)  [unwired: 2 in, 1 out]
        n267 = local read "Baseline Y"() -> (w388:dbl[])
        n268 = Subtract(x=w390, y=w388) -> (x-y=w387:dbl[])
      }
    }
    n269 = local read "Good NMR X"() -> (w121:dbl[])
    n270 = Or(x="Record All\nSweep Sets", y="Record Next \nSweep Set") -> (x .or. y?=w122:bool)
    "Recording" <- w122
    n271 = local read "Additive NMR Y"() -> (w116:dbl[])
    n272 = local read "Good NMR X"() -> (w115:dbl[])
    n273 = call "Convert to Dynamic Data28"("Array"=w121) -> ("Dynamic Data Type"=w120:dynamicdata)  [unwired: 3 in]
    n274 = call "Convert to Dynamic Data29"("Array"=w113) -> ("Dynamic Data Type"=w119:dynamicdata)  [unwired: 3 in]
    n275 = call "Convert to Dynamic Data12"("Array"=w67) -> ("Dynamic Data Type"=w26:dynamicdata)  [unwired: 3 in]
    "Modulator" <- w26
    n276 = case "Output Data to File" shown="True" w122 {
      tunnel: w166 -> [_ w428]
      tunnel: w116 -> [_ w435]
      tunnel: w115 -> [_ w434]
      frame False {
      }
      frame True {
        w400 = ";"
        n277 = call "Convert to Dynamic Data30"("Array"=w435) -> ("Dynamic Data Type"=w409:dynamicdata)  [unwired: 3 in]
        n278 = call "Convert to Dynamic Data32"("Array"=w434) -> ("Dynamic Data Type"=w408:dynamicdata)  [unwired: 3 in]
        n279 = local read "Up/Down Ave Y Final"() -> (w405:dbl[])
        n280 = local read "Baseline Subtract"() -> (w430:bool)
        n281 = local read "Number of Total\nSweeps Added"() -> (w436:i32)
        n282 = local read "Up/Down Ave X"() -> (w403:dbl[])
        n283 = local read "Use Wing Fit"() -> (w396:bool)
        n284 = local read "Baseline Y"() -> (w433:dbl[])
        n285 = local read "Triangle Wave\nRate (Hz)"() -> (w431:dbl)
        n286 = local read "Wing Fit"() -> (w401:dbl[])
        n287 = Boolean To (0,1)(Boolean=w430) -> (0, 1=w429:i16)
        n288 = Boolean To (0,1)(Boolean=w396) -> (0, 1=w397:i16)
        n289 = call "Convert to Dynamic Data11"("Array"=w433) -> ("Dynamic Data Type"=w432:dynamicdata)  [unwired: 3 in]
        n290 = call "Convert to Dynamic Data13"("Array"=w401) -> ("Dynamic Data Type"=w412:dynamicdata)  [unwired: 3 in]
        n291 = call "Convert to Dynamic Data36"("Array"=w403) -> ("Dynamic Data Type"=w402:dynamicdata)  [unwired: 3 in]
        n292 = call "Convert to Dynamic Data14"("Array"=w405) -> ("Dynamic Data Type"=w404:dynamicdata)  [unwired: 3 in]
        n293 = local read "Time of Last Baseline"() -> (w417:string)
        n294 = xnode "Set Dynamic Data Attributes"("Signals In"=w409) -> ("Signals Out"=w437:dynamicdata)  [unwired: 4 in, 1 out]
        n295 = xnode "Set Dynamic Data Attributes"("Signals In"=w432) -> ("Signals Out"=w411:dynamicdata)  [unwired: 4 in, 1 out]
        n296 = xnode "Set Dynamic Data Attributes"("Signals In"=w412) -> ("Signals Out"=w410:dynamicdata)  [unwired: 4 in, 1 out]
        n297 = xnode "Set Dynamic Data Attributes"("Signals In"=w402) -> ("Signals Out"=w406:dynamicdata)  [unwired: 4 in, 1 out]
        n298 = xnode "Set Dynamic Data Attributes"("Signals In"=w404) -> ("Signals Out"=w407:dynamicdata)  [unwired: 4 in, 1 out]
        n299 = xnode "Set Dynamic Data Attributes"("Signals In"=w408) -> ("Signals Out"=w439:dynamicdata)  [unwired: 4 in, 1 out]
        n300 = local read "Comment"() -> (w426:string)
        n301 = Number To Decimal String(number=w429) -> (decimal integer string=w422:string)  [unwired: 1 in]
        n302 = Number To Decimal String(number=w397) -> (decimal integer string=w398:string)  [unwired: 1 in]
        n303 = Number To Fractional String(number=w431) -> (F-format string=w420:string)  [unwired: 3 in]
        n304 = Number To Decimal String(number=w436) -> (decimal integer string=w424:string)  [unwired: 1 in]
        n305 = Concatenate Strings(w400, "Baseline Subtracted = ", w422, w400, "Time of Last Baseline = ", w417, w400, "Use Wing Fit = ", w398) -> (w416:string)
        n306 = Merge Signals(w439, w437, w411, w410, w406, w407) -> (w438:dynamicdata)
        n307 = Concatenate Strings(w428, w400, "User comment =  ", w426) -> (w419:string)
        n308 = Concatenate Strings(w400, "Triangle Wave Rate (Hz) = ", w420) -> (w415:string)
        n309 = Concatenate Strings(w400, "# of Sweeps = ", w424) -> (w414:string)
        n310 = Concatenate Strings(w419, w416, w415, w414) -> (w413:string)
        n311 = call "Write to File"("Signals"=w438, "Comment"=w413) -> ()  [unwired: 15 in, 3 out]
        "Time of Last Recording" <- w428
      }
    }
    n312 = call "Build XY Graph2"("Y Input"=w119, "X Input"=w120) -> ("XY Graph"=→"NMR":cluster{"Y":dbl[], "Y":dbl[]}[])  [unwired: 8 in, 1 out]
    n313 = call "Convert to Dynamic Data31"("Array"=w115) -> ("Dynamic Data Type"=w114:dynamicdata)  [unwired: 3 in]
    n314 = call "Build XY Graph"("error in (no error)"=w169, "Y Input"=w26, "X Input"=w114) -> ("XY Graph"=→"NMR":cluster{"Y":dbl[], "Y":dbl[]}[])  [unwired: 7 in, 1 out]
    n315 = case shown="True" "Use Wing Fit" {
      tunnel: w39 -> [w182 w184]
      tunnel: [w182 w183] -> w38
      frame False {
      }
      frame True {
        n316 = local read "Wing Fit"() -> (w185:dbl[])
        n317 = Subtract(x=w184, y=w185) -> (x-y=w183:dbl[])
      }
    }
    "Up/Down Ave Y Final" <- w38
    n318 = Divide(x="Peak Size", y=100.0) -> (x/y=w54:dbl)
    n319 = Multiply(x=500.0, y=w54) -> (x*y=w48:dbl)
    n320 = Divide(x=w48, y=2.0) -> (x/y=w50:dbl)
    n321 = call "Convert from Dynamic Data10"("Dynamic Data Type"=w94) -> ("Array"=w88:dbl[])  [unwired: 3 in]
    n322 = Subtract(x=250.0, y=w50) -> (x-y=w49:dbl)
    n323 = To Long Integer(number=w49) -> (32bit integer=w47:i32)
    n324 = To Long Integer(number=w48) -> (32bit integer=w46:i32)
    n325 = Array Subset(array=w88, index=w78, length=w77) -> (w45:dbl[])
    "Up/Down Ave X" <- w45
    n326 = call "Convert to Dynamic Data35"("Array"=w38) -> ("Dynamic Data Type"=w59:dynamicdata)  [unwired: 3 in]
    n327 = Array Subset(array=w38, index=w47, length=w46) -> (w42:dbl[])
    n328 = Array Subset(array=w45, index=w47, length=w46) -> (w44:dbl[])
    n329 = call "Convert to Dynamic Data34"("Array"=w45) -> ("Dynamic Data Type"=w62:dynamicdata)  [unwired: 3 in]
    n330 = call <vilib>:"Gaussian Peak Fit.vi"("Y"=w42, "X"=w44) -> ("Best Gaussian Fit"=w58:dbl[], "center"=→"Centroid:":dbl)  [unwired: 7 in, 5 out]
    n331 = call "Convert to Dynamic Data39"("Array"=w44) -> ("Dynamic Data Type"=w43:dynamicdata)  [unwired: 3 in]
    n332 = Merge Signals(w62, w43) -> (w61:dynamicdata)
    n333 = call "Convert to Dynamic Data38"("Array"=w58) -> ("Dynamic Data Type"=w57:dynamicdata)  [unwired: 3 in]
    n334 = Merge Signals(w59, w57) -> (w60:dynamicdata)
    n335 = call "Build XY Graph3"("Y Input"=w60, "X Input"=w61) -> ("XY Graph"=→"NMR":cluster{"Y":dbl[], "Y":dbl[]}[])  [unwired: 8 in, 1 out]
    "Baseline\nSubtract" <- "Baseline Subtract"
  }
  n336 = while "Comment Manager" {
    shift-right: [w668] -> _
    shift-left: _ -> [w671]
    stop <- "Heartbeat" stop-if-true
    n337 = Not(x=w671) -> (.not. x?=w668:bool)
    "Heartbeat" <- w668
    n338 = Get Date/Time In Seconds() -> (seconds since 1Jan1904=w666:timestamp)
    n339 = call "Time Delay"("Delay Time (s)"=1) -> ()  [unwired: 10 in, 1 out]
    n340 = case shown="False" "Submit" {
      frame False {
      }
      frame True {
      }
    }
    n341 = case shown="False" "Clear" {
      frame False {
      }
      frame True {
        n342 = local write "Comment"("") -> ()
      }
    }
    n343 = Get Date/Time String(seconds (now)=w666, want seconds? (F)=TRUE) -> (date string=w665:string, time string=w663:string)  [unwired: 1 in]
    n344 = Concatenate Strings(w665, " ", w663) -> (→"Lab Time":string)
  }
  n345 = while "Error Display" {
    stop <- "Error Beat" stop-if-true
    n346 = local read "Most Recent Error (Temp)"() -> (w673:string)
    n347 = local read "Most Recent Error (NMR)"() -> (w674:string)
    n348 = local read "Temp"() -> (w682:bool)
    n349 = local read "NMR"() -> (w681:bool)
    n350 = Or(x=w682, y=w681) -> (x .or. y?=w679:bool)
    n351 = Not(x="Silence Flashing") -> (.not. x?=w677:bool)
    n352 = And(x=w679, y=w677) -> (x .and. y?=w676:bool)
    "Is Flashing" <- w676
    n353 = case shown="True" w676 {
      frame False {
        n354 = local write "Errors"(FALSE) -> ()
      }
      frame True {
        n355 = while {
          shift-right: [w693] -> _
          shift-left: _ -> [w695]
          stop <- w692 stop-if-true
          n356 = local read "i"() -> (w686:dbl)
          n357 = Equal To 0?(x=w686) -> (x = 0?=w689:bool)
          n358 = Not(x=w695) -> (.not. x?=w693:bool)
          "Errors" <- w693
          n359 = Quotient & Remainder(x=w686, y=10) -> (x-y*floor(x/y)=w690:dbl)  [unwired: 1 out]
          n360 = Equal To 0?(x=w690) -> (x = 0?=w688:bool)
          n361 = call "Time Delay3"("Delay Time (s)"=0.3) -> ()  [unwired: 10 in, 1 out]
          n362 = Or(x=w689, y=w688) -> (x .or. y?=w687:bool)
          n363 = Add(x=w686, y=1.0) -> (x+y=→"i":dbl)
          n364 = local read "Is Flashing"() -> (w692:bool)
          n365 = case shown="True" w687 {
            frame False {
            }
            frame True {
              n366 = call "Error Beep.vi"() -> ()  [unwired: 12 in]
            }
          }
        }
      }
    }
    n367 = Concatenate Strings(w673, w674) -> (→"Most Recent Error":string)
  }
  n368 = Get Date/Time In Seconds() -> (seconds since 1Jan1904=w24:timestamp)
  n369 = while "Temperature System" {
    stop <- "Temp Strip Chart" stop-if-true
    w773 = ";"
    w802 = 999999.0
    w817 = "R"
    w818 = "SIG:RES:"
    w824 = "SIG:TEMP:"
    w823 = "K"
    n370 = Divide(x="Time Between\nTemp Ponts (s)", y=2.0) -> (x/y=w792:dbl)
    n371 = call-poly <instrlib>:"Open.vi"("VISA resource name"="VISA resource name") -> ("error out"=w731:errorcluster, "Mercury Reference Out"=w729:T2)  [unwired: 6 in, 3 out]
    n372 = call "Instrument I/O Assistant - iTC - T"("error in"=w731) -> ("AB1.T"=w822:string, "CCS.T"=w827:string, "Pill.T"=w830:string, "error out"=w734:errorcluster)  [unwired: 22 in, 1 out]
    n373 = call "Time Delay2"("error in (no error)"=w734, "Delay Time (s)"=w792) -> ("error out"=w797:errorcluster)  [unwired: 9 in]
    n374 = call "Instrument I/O Assistant - iTC - R"("error in"=w797) -> ("AB1.R"=w794:string, "CCS.R"=w795:string, "Pill.R"=w796:string, "error out"=w730:errorcluster)  [unwired: 22 in, 1 out]
    n375 = Match Pattern(string=w794, regular expression=w818) -> (after substring=w814:string)  [unwired: 1 in, 3 out]
    n376 = Match Pattern(string=w795, regular expression=w818) -> (after substring=w816:string)  [unwired: 1 in, 3 out]
    n377 = Match Pattern(string=w796, regular expression=w818) -> (after substring=w815:string)  [unwired: 1 in, 3 out]
    n378 = Match Pattern(string=w814, regular expression=w817) -> (before substring=w811:string)  [unwired: 1 in, 3 out]
    n379 = Match Pattern(string=w816, regular expression=w817) -> (before substring=w813:string)  [unwired: 1 in, 3 out]
    n380 = Match Pattern(string=w815, regular expression=w817) -> (before substring=w812:string)  [unwired: 1 in, 3 out]
    n381 = call <instrlib>:"Close.vi"("error in (no error)"=w730, "Mercury Reference"=w729) -> ("error out"=w721:errorcluster)  [unwired: 9 in]
    n382 = Match Pattern(string=w830, regular expression=w824) -> (after substring=w829:string)  [unwired: 1 in, 3 out]
    n383 = Match Pattern(string=w827, regular expression=w824) -> (after substring=w826:string)  [unwired: 1 in, 3 out]
    n384 = Match Pattern(string=w822, regular expression=w824) -> (after substring=w821:string)  [unwired: 1 in, 3 out]
    n385 = To Long Integer(number="AB2/3/4 Switch") -> (32bit integer=w742:i32)
    n386 = Scan String For Tokens(9:w811) -> (1:w808:string)  [unwired: 5 in, 3 out]
    n387 = Scan String For Tokens(9:w813) -> (1:w810:string)  [unwired: 5 in, 3 out]
    n388 = Scan String For Tokens(9:w812) -> (1:w809:string)  [unwired: 5 in, 3 out]
    n389 = call "Instrument I/O Assistant - Fluke MM"() -> ("AB3.R"=w749:dbl, "error out"=w800:errorcluster)  [unwired: 25 in, 1 out]
    n390 = Match Pattern(string=w829, regular expression=w823) -> (before substring=w828:string)  [unwired: 1 in, 3 out]
    n391 = Match Pattern(string=w826, regular expression=w823) -> (before substring=w825:string)  [unwired: 1 in, 3 out]
    n392 = Match Pattern(string=w821, regular expression=w823) -> (before substring=w820:string)  [unwired: 1 in, 3 out]
    n393 = Fract/Exp String To Number(string=w808) -> (number=w803:dbl)  [unwired: 3 in, 1 out]
    n394 = Fract/Exp String To Number(string=w810) -> (number=w783:dbl)  [unwired: 3 in, 1 out]
    n395 = Fract/Exp String To Number(string=w809) -> (number=w804:dbl)  [unwired: 3 in, 1 out]
    n396 = Add(x=w742, y=2) -> (x+y=→"AB" →"AB   .T":i32)
    n397 = Equal?(x=1, y=w742) -> (x = y?=w751:bool)
    n398 = Equal?(x=0, y=w742) -> (x = y?=w752:bool)
    n399 = Equal?(x=2, y=w742) -> (x = y?=w750:bool)
    n400 = call "Instrument I/O Assistant - iTC - T3"() -> ("AB4.R"=w700:dbl, "AB4.T"=w696:dbl, "AB3.R"=w719:dbl, "AB3.T"=w701:dbl, "AB2.R"=w725:dbl, "AB2.T"=w702:dbl, "error out"=w720:errorcluster)  [unwired: 20 in, 1 out]
    n401 = Greater?(x=w803, y=w802) -> (0:w717:bool)
    n402 = Greater?(x=w749, y=w802) -> (0:w801:bool)
    n403 = Greater?(x=w783, y=w802) -> (0:w715:bool)
    n404 = Greater?(x=w804, y=w802) -> (0:w716:bool)
    n405 = Scan String For Tokens(9:w828) -> (1:w841:string)  [unwired: 5 in, 3 out]
    n406 = Scan String For Tokens(9:w825) -> (1:w839:string)  [unwired: 5 in, 3 out]
    n407 = Scan String For Tokens(9:w820) -> (1:w838:string)  [unwired: 5 in, 3 out]
    n408 = Less?(x=w749, y=0.1) -> (x < y?=→"Fluke Err":bool)
    n409 = case shown="True" w750 {
      tunnel: w749 -> [_ w943]
      tunnel: [w941 w943] -> _
      tunnel: [w941 w942] -> _
      frame False {
        w941 = 0.0
      }
      frame True {
        n410 = formula code="T=1/(-0.2209+0.0454036*ln(R));" "AB4 Calibration"("R"=w943) -> ("T"=w942:dbl)
      }
    }
    n411 = local read "Reset iTC"() -> (w733:bool)
    n412 = case shown="True" w752 {
      tunnel: w749 -> [_ w949]
      tunnel: [w947 w949] -> _
      tunnel: [w947 w948] -> _
      frame False {
        w947 = 0.0
      }
      frame True {
        n413 = formula code="T=1/(-0.37015159+0.07857834*ln(R)+0.0/ln(R));" "AB2 Calibration"("R"=w949) -> ("T"=w948:dbl)
      }
    }
    n414 = case shown="False" w733 {
      frame False {
        n415 = local read "iTC Last Reset"() -> (w847:timestamp)
        n416 = Get Date/Time In Seconds() -> (seconds since 1Jan1904=w848:timestamp)
        n417 = Subtract(x=w848, y=w847) -> (x-y=w846:dbl)
        n418 = Divide(x=w846, y=60.0) -> (x/y=w844:dbl)
        "Time Since iTC Reset\n(min)" <- w844
        n419 = Greater Or Equal?(x=w844, y="Time b/t iTC Resets\n(min)") -> (x >= y?=w842:bool)
        n420 = local write "Reset iTC"(w842) -> ()
      }
      frame True {
        n421 = call "Instrument I/O Assistant - iTC - T2"() -> ()  [unwired: 25 in, 3 out]
        n422 = Get Date/Time In Seconds() -> (seconds since 1Jan1904=→"iTC Last Reset":timestamp)
        "Reset iTC" <- FALSE
      }
    }
    n423 = Fract/Exp String To Number(string=w841) -> (number=w699:dbl)  [unwired: 3 in, 1 out]
    "?" <- w699
    n424 = Fract/Exp String To Number(string=w839) -> (number=w704:dbl)  [unwired: 3 in, 1 out]
    "?" <- w704
    n425 = Equal To 0?(x=w704) -> (x = 0?=w726:bool)
    n426 = Fract/Exp String To Number(string=w838) -> (number=w703:dbl)  [unwired: 3 in, 1 out]
    "?" <- w703
    n427 = Equal To 0?(x=w703) -> (x = 0?=w727:bool)
    n428 = Equal To 0?(x=w699) -> (x = 0?=w728:bool)
    n429 = Build Array(w715, w716, w717, w801, w728, w727, w726) -> (w806:bool[])
    n430 = local read "Baseline Subtracted Integral vs. Time"() -> (w782:dbl)
    n431 = local read "Vapor Pressure\n(mTorr)"() -> (w768:dbl)
    n432 = Or Array Elements(Boolean array=w806) -> (logical OR=w805:bool)
    n433 = local read "V.P. Temp\n(K)"() -> (w697:dbl)
    n434 = local read "Flow (SLM)"() -> (w738:dbl)
    n435 = case "Error Handler - Fluke MM Resistor Value" shown="True" w805 {
      tunnel: [w1022 w1027] -> w799
      frame False {
        n436 = call <vilib>:"General Error Handler.vi"("[error code] (0)"=0) -> ("error out"=w1022:errorcluster)  [unwired: 10 in, 4 out]
      }
      frame True {
        n437 = call <vilib>:"General Error Handler.vi"("[error code] (0)"=5042, "[error source] (\" \")"="Thermistor Value", "type of dialog (OK msg:1)"=0) -> ("error out"=w1027:errorcluster)  [unwired: 8 in, 4 out]
      }
    }
    n438 = call "Convert to Dynamic Data2"("Double"=w704) -> ("Dynamic Data Type"=w712:dynamicdata)  [unwired: 3 in]
    "CCS.T" <- w712
    n439 = call "Convert to Dynamic Data3"("Double"=w703) -> ("Dynamic Data Type"=w711:dynamicdata)  [unwired: 3 in]
    "AB1.T" <- w711
    n440 = call "Convert to Dynamic Data4"("Double"=w783) -> ("Dynamic Data Type"=w756:dynamicdata)  [unwired: 3 in]
    "CCS.R" <- w756
    n441 = call "Convert to Dynamic Data5"("Double"=w804) -> ("Dynamic Data Type"=w758:dynamicdata)  [unwired: 3 in]
    "AB5.R" <- w758
    n442 = call "Convert to Dynamic Data6"("Double"=w803) -> ("Dynamic Data Type"=w757:dynamicdata)  [unwired: 3 in]
    "AB1.R" <- w757
    n443 = call "Convert to Dynamic Data"("Double"=w699) -> ("Dynamic Data Type"=w707:dynamicdata)  [unwired: 3 in]
    "AB5.T" <- w707
    n444 = local read "Q Meter Temp"() -> (w706:dynamicdata)
    n445 = case shown="True" w751 {
      tunnel: w749 -> [_ w946]
      tunnel: [w944 w946] -> _
      tunnel: [w944 w945] -> _
      frame False {
        w944 = 0.0
      }
      frame True {
        n446 = formula code="T=1/(-0.18336724+0.0371466*ln(R)+0.0/ln(R));" "AB3 Calibration"("R"=w946) -> ("T"=w945:dbl)
      }
    }
    n447 = call "Convert to Dynamic Data19"("Double"=w768) -> ("Dynamic Data Type"=→"Vapor Pressure":dynamicdata)  [unwired: 3 in]
    n448 = call "Convert to Dynamic Data21"("Double"=w719) -> ("Dynamic Data Type"=w713:dynamicdata)  [unwired: 3 in]
    "AB3.R" <- w713
    n449 = call "Convert to Dynamic Data22"("Double"=w701) -> ("Dynamic Data Type"=w709:dynamicdata)  [unwired: 3 in]
    "AB3.T" <- w709
    n450 = call "Convert to Dynamic Data16"("Double"=w782) -> ("Dynamic Data Type"=w781:dynamicdata)  [unwired: 3 in]
    n451 = call "Convert to Dynamic Data17"("Double"=w768) -> ("Dynamic Data Type"=w772:dynamicdata)  [unwired: 3 in]
    n452 = call "Convert to Dynamic Data25"("Double"=w725) -> ("Dynamic Data Type"=w722:dynamicdata)  [unwired: 3 in]
    "AB2.R" <- w722
    n453 = call "Convert to Dynamic Data26"("Double"=w702) -> ("Dynamic Data Type"=w710:dynamicdata)  [unwired: 3 in]
    "AB2.T" <- w710
    n454 = call "Convert to Dynamic Data23"("Double"=w700) -> ("Dynamic Data Type"=w714:dynamicdata)  [unwired: 3 in]
    "AB4.R" <- w714
    n455 = call "Convert to Dynamic Data24"("Double"=w696) -> ("Dynamic Data Type"=w708:dynamicdata)  [unwired: 3 in]
    "AB4.T" <- w708
    n456 = call "Convert to Dynamic Data27"("Double"=w738) -> ("Dynamic Data Type"=w737:dynamicdata)  [unwired: 3 in]
    n457 = Compound Arithmetic op=ADD(w725, w719, w700) -> (w739:dbl)
    "?" <- w739
    n458 = Compound Arithmetic op=ADD(w701, w696) -> (w740:dbl)
    n459 = call "Convert to Dynamic Data18"("Double"=w697) -> ("Dynamic Data Type"=w705:dynamicdata)  [unwired: 3 in]
    n460 = call "Convert from Dynamic Data5"("Dynamic Data Type"=w706) -> ("Scalar"=w698:dbl)  [unwired: 3 in]
    n461 = xnode "Set Dynamic Data Attributes"("Signals In"=w707) -> ("Signals Out"=w763:dynamicdata)  [unwired: 4 in, 1 out]
    n462 = xnode "Set Dynamic Data Attributes"("Signals In"=w712) -> ("Signals Out"=w764:dynamicdata)  [unwired: 4 in, 1 out]
    n463 = xnode "Set Dynamic Data Attributes"("Signals In"=w711) -> ("Signals Out"=w766:dynamicdata)  [unwired: 4 in, 1 out]
    n464 = xnode "Set Dynamic Data Attributes"("Signals In"=w756) -> ("Signals Out"=w762:dynamicdata)  [unwired: 4 in, 1 out]
    n465 = xnode "Set Dynamic Data Attributes"("Signals In"=w758) -> ("Signals Out"=w759:dynamicdata)  [unwired: 4 in, 1 out]
    n466 = xnode "Set Dynamic Data Attributes"("Signals In"=w757) -> ("Signals Out"=w761:dynamicdata)  [unwired: 4 in, 1 out]
    n467 = xnode "Set Dynamic Data Attributes"("Signals In"=w713) -> ("Signals Out"=w760:dynamicdata)  [unwired: 4 in, 1 out]
    n468 = xnode "Set Dynamic Data Attributes"("Signals In"=w709) -> ("Signals Out"=w765:dynamicdata)  [unwired: 4 in, 1 out]
    n469 = xnode "Set Dynamic Data Attributes"("Signals In"=w706) -> ("Signals Out"=w785:dynamicdata)  [unwired: 4 in, 1 out]
    n470 = xnode "Set Dynamic Data Attributes"("Signals In"=w781) -> ("Signals Out"=w780:dynamicdata)  [unwired: 4 in, 1 out]
    n471 = xnode "Set Dynamic Data Attributes"("Signals In"=w772) -> ("Signals Out"=w771:dynamicdata)  [unwired: 4 in, 1 out]
    n472 = xnode "Set Dynamic Data Attributes"("Signals In"=w705) -> ("Signals Out"=w770:dynamicdata)  [unwired: 4 in, 1 out]
    n473 = xnode "Set Dynamic Data Attributes"("Signals In"=w722) -> ("Signals Out"=w724:dynamicdata)  [unwired: 4 in, 1 out]
    n474 = xnode "Set Dynamic Data Attributes"("Signals In"=w710) -> ("Signals Out"=w723:dynamicdata)  [unwired: 4 in, 1 out]
    n475 = xnode "Set Dynamic Data Attributes"("Signals In"=w714) -> ("Signals Out"=w748:dynamicdata)  [unwired: 4 in, 1 out]
    n476 = xnode "Set Dynamic Data Attributes"("Signals In"=w708) -> ("Signals Out"=w747:dynamicdata)  [unwired: 4 in, 1 out]
    n477 = xnode "Set Dynamic Data Attributes"("Signals In"=w737) -> ("Signals Out"=w736:dynamicdata)  [unwired: 4 in, 1 out]
    n478 = call "Convert to Dynamic Data8"("Double"=w740) -> ("Dynamic Data Type"=→"AB2/3/4.T":dynamicdata)  [unwired: 3 in]
    n479 = Merge Signals(w763, w764, w766, w762, w759, w761, w760, w765, w785, w780, w771, w770, w724, w723, w748, w747, w736) -> (w832:dynamicdata)
    n480 = call "Convert to Dynamic Data7"("Double"=w739) -> ("Dynamic Data Type"=→"AB2/3/4.R":dynamicdata)  [unwired: 3 in]
    n481 = Get Date/Time In Seconds() -> (seconds since 1Jan1904=w837:timestamp)
    n482 = Build Array(w720, w721, w800, w799) -> (w798:errorcluster[])
    n483 = Get Date/Time String(seconds (now)=w837, want seconds? (F)=TRUE) -> (date string=w835:string, time string=w833:string)  [unwired: 1 in]
    n484 = Merge Errors(w798) -> (w807:errorcluster)
    n485 = local read "Comment"() -> (w790:string)
    n486 = Concatenate Strings(w835, " ", w833) -> (w786:string)
    n487 = Not(x="Ignore \nErrors") -> (.not. x?=w779:bool)
    n488 = call <vilib>:"General Error Handler.vi"("type of dialog (OK msg:1)"=0, "error in (no error)"=w807) -> ("error?"=w778:bool, "source out"=w787:string, "message"=w789:string)  [unwired: 9 in, 2 out]
    n489 = Select(t="Temperature Errors Ignored", s="Ignore \nErrors", f="") -> (s? t:f=w774:string)
    n490 = And(x=w779, y=w778) -> (x .and. y?=w753:bool)
    "Temp" <- w753
    "Temp" <- w753
    "Temp" <- w753
    n491 = Concatenate Strings(w786, w773, "User comment =  ", w790, w773, w789, w773, w787, w773, w774) -> (w788:string)
    n492 = case shown="False" w753 {
      tunnel: w704 -> [w1130 _]
      tunnel: w703 -> [w1129 _]
      tunnel: w702 -> [w1128 _]
      tunnel: w701 -> [w1127 _]
      tunnel: w696 -> [w1126 _]
      tunnel: w699 -> [w1125 _]
      tunnel: w698 -> [w1124 _]
      tunnel: w697 -> [w1123 _]
      frame False {
        n493 = Merge Signals(w1130, w1129, w1128, w1127, w1126, w1125, w1124, w1123) -> (→"Temperature Strip Chart":dynamicdata)
      }
      frame True {
        n494 = call "Instrument I/O Assistant - iTC - IFC"() -> ()  [unwired: 23 in, 5 out]
      }
    }
    n495 = case shown="True" w753 {
      tunnel: w804 -> [w1122 _]
      tunnel: w783 -> [w1121 _]
      tunnel: w803 -> [w1120 _]
      tunnel: w749 -> [w1119 _]
      frame False {
        n496 = Merge Signals(w1122, w1121, w1120, w1119) -> (→"Resistance Strip Chart":dynamicdata)
      }
      frame True {
      }
    }
    n497 = case shown="True" w753 {
      tunnel: w832 -> [w1134 w1137]
      tunnel: w788 -> [w1133 w1136]
      tunnel: [w1132 w1135] -> w819
      frame False {
        n498 = call "Write To Measurement File"("Signals"=w1134, "Comment"=w1133) -> ("error out"=w1132:errorcluster)  [unwired: 15 in, 2 out]
      }
      frame True {
        n499 = call "Write to Error File"("Signals"=w1137, "Comment"=w1136) -> ("error out"=w1135:errorcluster)  [unwired: 15 in, 2 out]
      }
    }
    n500 = case shown="True" w753 {
      tunnel: w788 -> [w1192 w1193]
      frame False {
        "Last Measurement Taken" <- w1192
      }
      frame True {
        "Most Recent Error (Temp)" <- w1193
      }
    }
    n501 = call "Time Delay"("error in (no error)"=w819, "Delay Time (s)"=w792) -> ()  [unwired: 9 in, 1 out]
  }
  n502 = Initialize Array(0.0, 1000) -> (→"Baseline Y":dbl[])
  n503 = Initialize Array(0.0, 1000) -> (→"NMR X Check":dbl[])
  n504 = Initialize Array(0.0, 1000) -> (→"Baseline X":dbl[])
  n505 = Initialize Array(0.0, 1000) -> (→"Good NMR X":dbl[])
  n506 = Initialize Array(0.0, 1000) -> (→"Additive NMR Y":dbl[])
  n507 = Initialize Array(0.0, 1000) -> (→"Zeroed Array":dbl[])
  n508 = Get Date/Time String(seconds (now)=w24, want seconds? (F)=TRUE) -> (date string=w23:string, time string=w21:string)  [unwired: 1 in]
  n509 = Concatenate Strings(w23, " ", w21) -> (→"VI Start Time":string)
  "Just Started" <- TRUE
